vi "calcUpdatePeriod.vi"(8 "error in (no error)":errorcluster, 11 "ILC in":refnum<class "ILC.lvclass">) -> (0 "error out":errorcluster, 3 "ILC out":refnum<class "ILC.lvclass">)   [LabVIEW 2015, in "ILCCommon.lvlib" / "ILC.lvclass"]
uses:
  <userlib>/Common/ILC/ILC/ILC.lvclass
  <userlib>/Common/ILC/ILC/ILC.lvclass/ILC.ctl
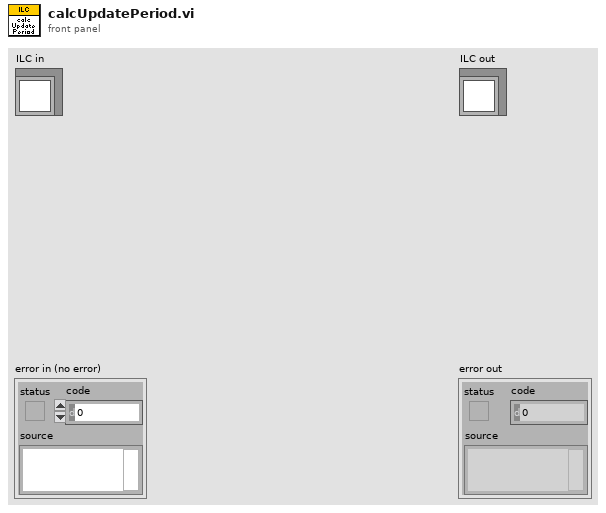
[diagram p1: front panel]
types:
  T1 = typedef "ILCCommon.lvlib/ILCConfiguration.lvlib/Input Channels.ctl" = enum16{"Channel 0", "3 Channels", "5 Channels"}
  T2 = typedef "ILCCommon.lvlib/ILCConfiguration.lvlib/Scan Rates.ctl" = enum16{"50", "60", "100", "120", "200", "240", "300", "400", "480", "600", "1200", "2400", "4800"}
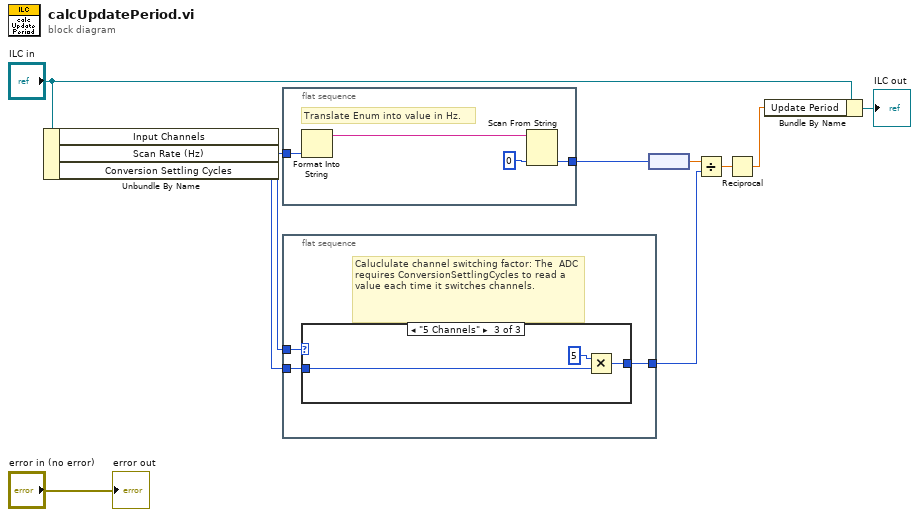
[diagram p0: block diagram]
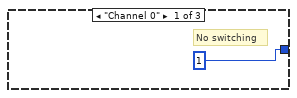
[diagram p2: hidden frame]
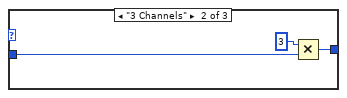
[diagram p3: hidden frame]
diagram:
  n1 = Unbundle By Name("ILC in") -> ("Input Channels"=w10:T1, "Scan Rate (Hz)"=w9:T2, "Conversion Settling Cycles"=w2:u16)
  n2 = flat-sequence {
    tunnel: w9 -> [w13]
    tunnel: [w12] -> w8
    frame #0 {
      # "Translate Enum into value in Hz."
      n3 = Format Into String(w13) -> (resulting string=w14:string)  [unwired: 3 in, 1 out]
      n4 = Scan From String(input string=w14, default 1=u16 0 ("Numeric")) -> (output 1=w12:u16)  [unwired: 3 in, 3 out]
    }
  }
  n5 = flat-sequence {
    tunnel: w10 -> [w18]
    tunnel: [w16] -> w7
    tunnel: w2 -> [w17]
    frame #0 {
      # "Caluclulate channel switching factor: The  ADC requires ConversionSettlingCycles to read a value each time it switches channels."
      n6 = case shown="\"5 Channels\"" w18 {
        tunnel: [u16 1 ("Numeric") w20 w23] -> w16
        tunnel: w17 -> [_ w21 w24]
        frame "Channel 0" {
          # "No switching"
        }
        frame "3 Channels" {
          n7 = Multiply(x=u16 3 ("Numeric"), y=w21) -> (x*y=w20:u16)
        }
        frame "5 Channels" {
          n8 = Multiply(x=u16 5 ("Numeric"), y=w24) -> (x*y=w23:u16)
        }
      }
    }
  }
  n9 = node(w8) -> (w1:dbl[unit])
  n10 = Divide(x=w1, y=w7) -> (x/y=w4:dbl[unit])
  n11 = Reciprocal(x=w4) -> (1/x=w3:dbl[unit])
  n12 = Bundle By Name(cluster="ILC in", "Update Period"=w3) -> (→"ILC out":refnum<class "ILC.lvclass">)
  "error out" <- "error in (no error)"
